vi "Init System.vi"(8 "error in (no error)":errorcluster, 11 "Windows System SAL in":refnum<class "Windows System SAL.lvclass">) -> (0 "error out":errorcluster, 3 "Windows System SAL out":refnum<class "Windows System SAL.lvclass">)   [LabVIEW 2020, in "Volatus.lvlib" / "Windows System SAL.lvclass"]
uses:
  Windows System SAL.lvclass
  Windows System SAL.lvclass/Windows System SAL.ctl
  <vilib>/nisyscfg/nisyscfg.lvlib
  <resource>/objmgr/nisysapi.rc
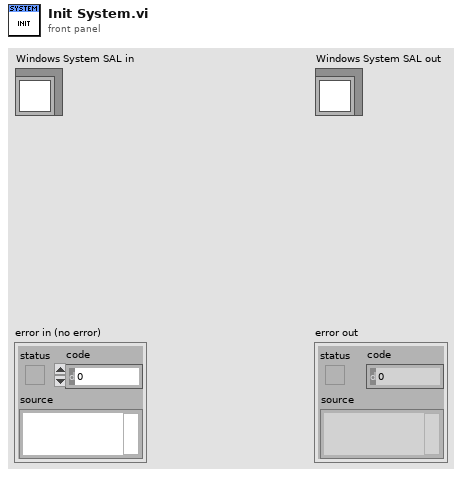
[diagram p1: front panel]
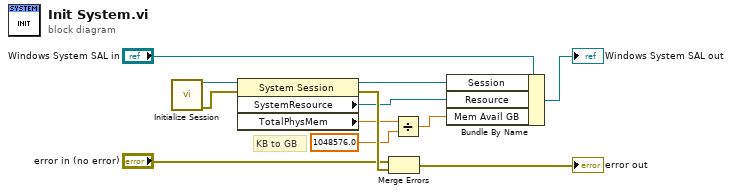
[diagram p0: block diagram]
diagram:
  # "KB to GB"
  n1 = call <vilib>:"Initialize Session.vi"() -> ("error out"=w8:errorcluster, "Session out"=w9:refnum<k21>)  [unwired: 10 in]
  n2 = property class="System Session"(reference=w9, error in=w8) -> (reference out=w6:refnum<k21>, error out=w12:errorcluster, "SystemResource"=w5:refnum<k20>, "TotalPhysMem"=w3:dbl)
  n3 = Merge Errors("error in (no error)", w12) -> (→"error out":errorcluster)
  n4 = Divide(x=w3, y=1048576.0) -> (x/y=w1:dbl)
  n5 = Bundle By Name(cluster="Windows System SAL in", "Session"=w6, "Resource"=w5, "Mem Avail GB"=w1) -> (→"Windows System SAL out":refnum<class "Windows System SAL.lvclass">)
